vi "Edit WaitMoniter.vi"(8 "error in":errorcluster, 10 "WaitMoniter Input":T2={"Wait Time(S)"=10.0, "Chamber Temp(Deg C)"=10.0, "Chamber Temp Tolerance(%)"=10.0, "RMS Current(A)"=10.0, "RMS Current Tolerance(%)"=10.0, "Temperature Control"=FALSE, "RMS Control"=FALSE, "RMS Current Min(A)"=10.0, "RMS Current Max(A)"=10.0, "Chamber Temp Min(Deg C)"=10.0, "Chamber Temp Max(Deg C)"=10.0, "HVPPS Current Max(A)"=10.0, "HVPPS Control"=FALSE, "HVPPS Current(A)"=10.0} {"HVPPS Current(A)" format="%#_13g"; "HVPPS Current Max(A)" format="%#_13g"; "Chamber Temp Max(Deg C)" format="%#_13g"; "Chamber Temp Min(Deg C)" format="%#_13g"; "RMS Current Max(A)" format="%#_13g"; "RMS Current Min(A)" format="%#_13g"; "RMS Current Tolerance(%)" format="%#_13g"; "RMS Current(A)" format="%#_13g"; "Chamber Temp Tolerance(%)" format="%#_13g"; "Chamber Temp(Deg C)" format="%#_13g"; "Wait Time(S)" format="%#_13g"}, 11 "Sequence Context In":refnum<k7>) -> (0 "error out":errorcluster, 2 "WaitMoniter Output":T2={"Wait Time(S)"=10.0, "Chamber Temp(Deg C)"=10.0, "Chamber Temp Tolerance(%)"=10.0, "RMS Current(A)"=10.0, "RMS Current Tolerance(%)"=10.0, "Temperature Control"=FALSE, "RMS Control"=FALSE, "RMS Current Min(A)"=10.0, "RMS Current Max(A)"=10.0, "Chamber Temp Min(Deg C)"=10.0, "Chamber Temp Max(Deg C)"=10.0, "HVPPS Current Max(A)"=10.0, "HVPPS Control"=FALSE, "HVPPS Current(A)"=10.0} {"HVPPS Current(A)" format="%#_13g"; "HVPPS Current Max(A)" format="%#_13g"; "Chamber Temp Max(Deg C)" format="%#_13g"; "Chamber Temp Min(Deg C)" format="%#_13g"; "RMS Current Max(A)" format="%#_13g"; "RMS Current Min(A)" format="%#_13g"; "RMS Current Tolerance(%)" format="%#_13g"; "RMS Current(A)" format="%#_13g"; "Chamber Temp Tolerance(%)" format="%#_13g"; "Chamber Temp(Deg C)" format="%#_13g"; "Wait Time(S)" format="%#_13g"})   [LabVIEW 2023, in "LTT_TeststandSteptypes.lvlib"]
uses:
  LTT_TeststandSteptypes.lvlib
  Control/Wait Monitor Control.ctl
  Control/Moniter Step Control.ctl
  <vilib>/addons/TestStand/_TSUtility.llb/TestStand - Start Modal Dialog (Sequence Context).vi
  <vilib>/addons/TestStand/_TSUtility.llb/TestStand - End Modal Dialog (Sequence Context).vi
  HardwareAbstractionLayer_LVOOP/Database/Database.lvclass
  HardwareAbstractionLayer_LVOOP/Database/SQL Public VI/Control/DB Options.ctl
  HardwareAbstractionLayer_LVOOP/Power Moniter/Wait Monitor_class/Wait Monitor.lvclass
panel:
  in  "WaitMoniter":T1={"Wait Time(S)"=10.0, "RMS Current Min(A)"=10.0, "Temperature Control"=FALSE, "RMS Control"=FALSE, "RMS Current Max(A)"=10.0, "Chamber Temp Min(Deg C)"=10.0, "Chamber Temp Max(Deg C)"=10.0} {"Chamber Temp Max(Deg C)" format="%#_13g"; "Chamber Temp Min(Deg C)" format="%#_13g"; "RMS Current Max(A)" format="%#_13g"; "RMS Current Min(A)" format="%#_13g"; "Wait Time(S)" format="%#_13g"}
  in  "Close":bool
  in  "OK":bool
  # "WAIT AND MONITOR"
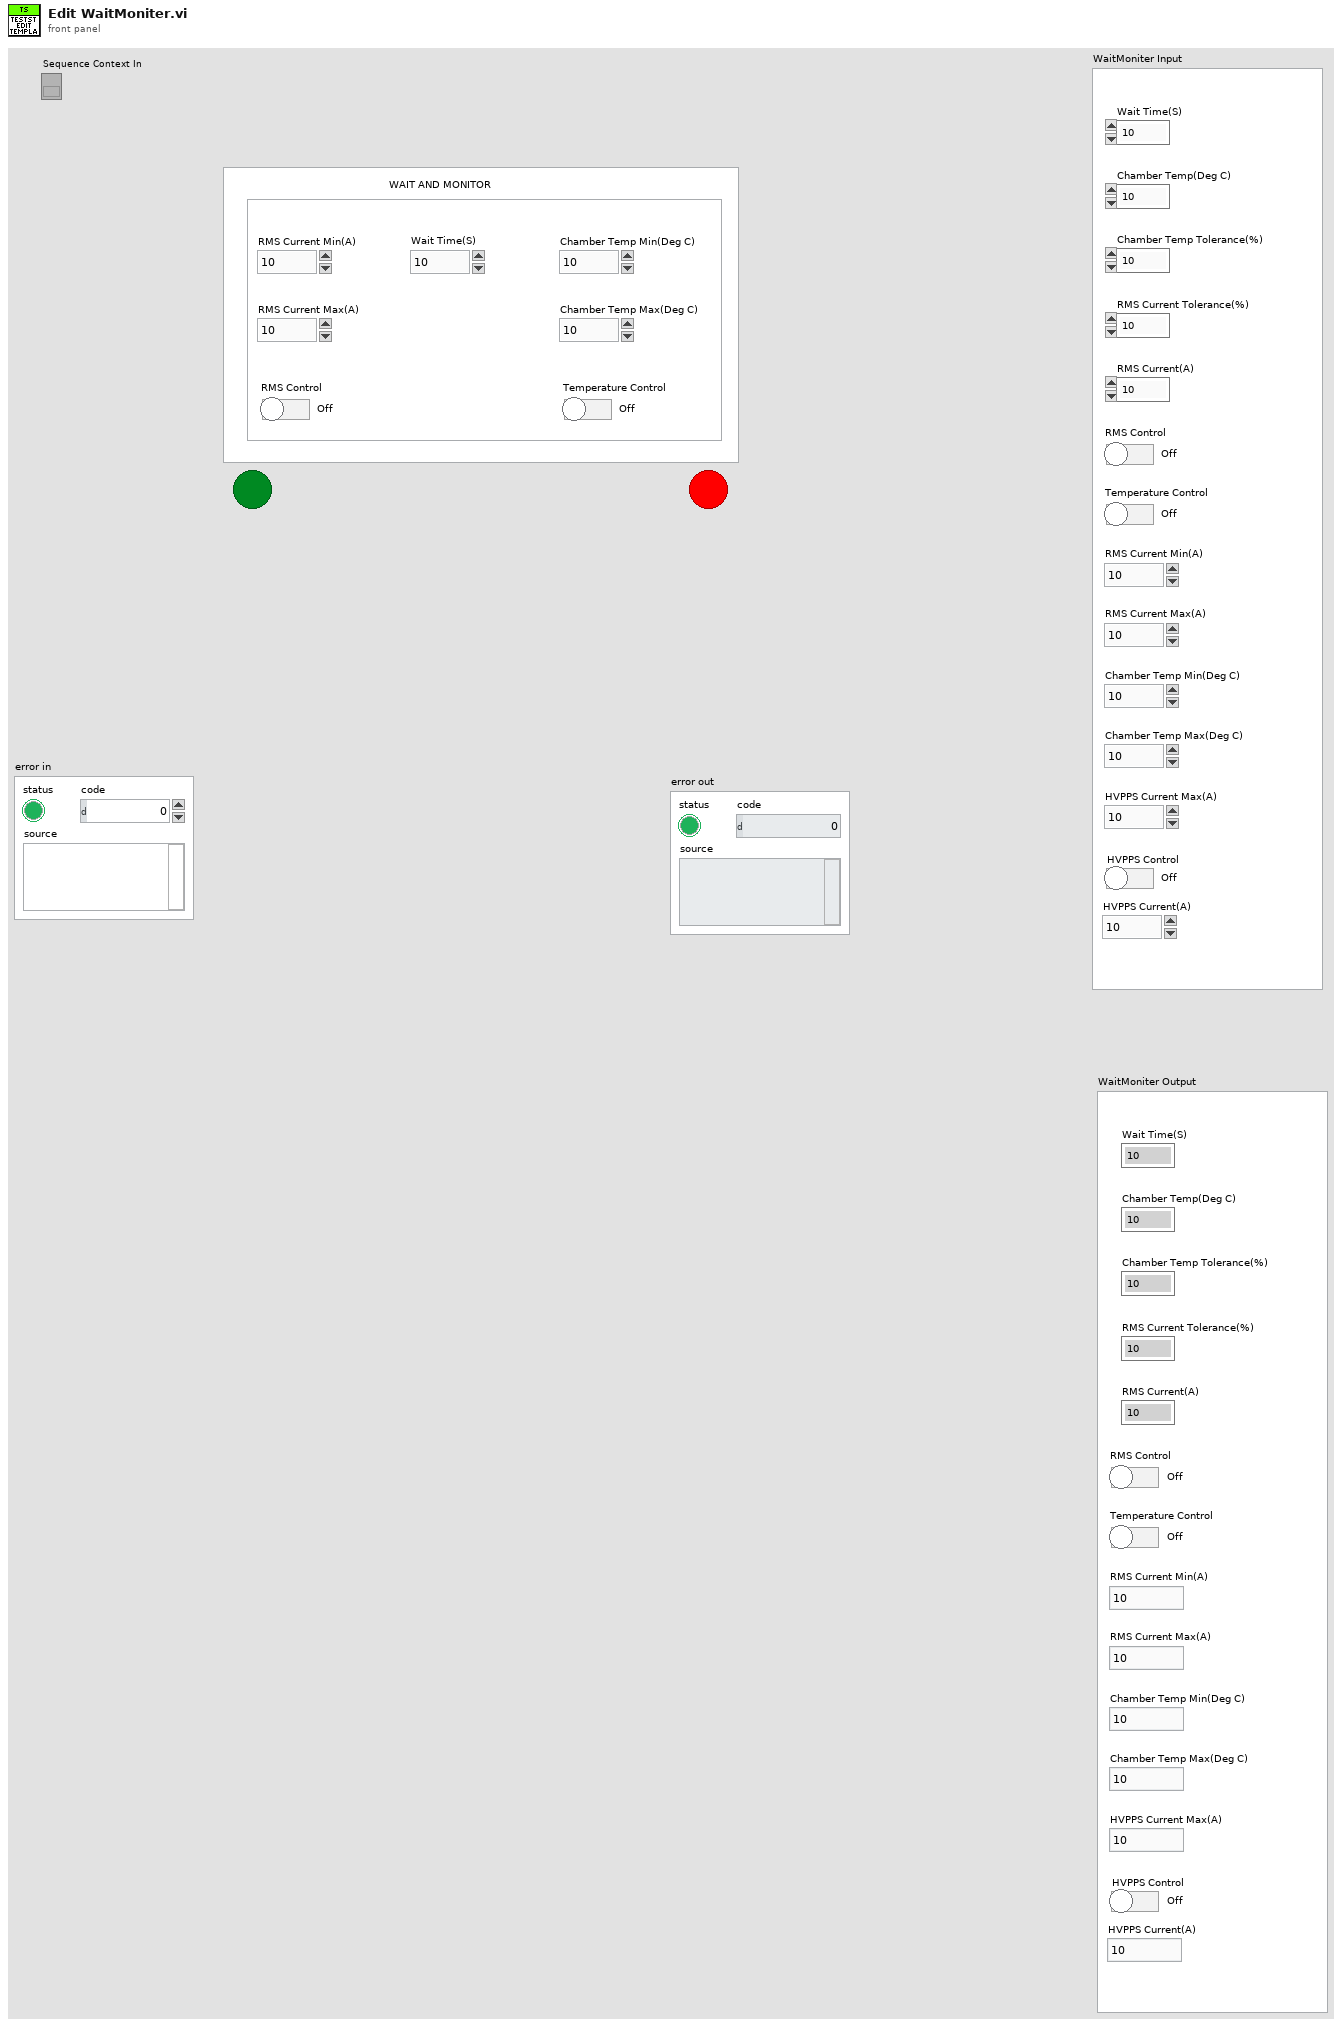
[diagram p1: front panel]
types:
  T1 = typedef "LTT_TeststandSteptypes.lvlib/Wait Monitor Control.ctl" = cluster{"Wait Time(S)":dbl, "RMS Current Min(A)":dbl, "Temperature Control":bool, "RMS Control":bool, "RMS Current Max(A)":dbl, "Chamber Temp Min(Deg C)":dbl, "Chamber Temp Max(Deg C)":dbl}
  T2 = typedef "HardwareAbstractionLayer_LVOOP.lvlib/Wait Monitor.lvclass/Moniter Step Control.ctl" = cluster{"Wait Time(S)":dbl, "Chamber Temp(Deg C)":dbl, "Chamber Temp Tolerance(%)":dbl, "RMS Current(A)":dbl, "RMS Current Tolerance(%)":dbl, "Temperature Control":bool, "RMS Control":bool, "RMS Current Min(A)":dbl, "RMS Current Max(A)":dbl, "Chamber Temp Min(Deg C)":dbl, "Chamber Temp Max(Deg C)":dbl, "HVPPS Current Max(A)":dbl, "HVPPS Control":bool, "HVPPS Current(A)":dbl}
  T3 = typedef "HardwareAbstractionLayer_LVOOP.lvlib/Database.lvclass/DB Options.ctl" = enum16{"Init", "Select Data", "Insert Data", "Update Data", "Delete Data", "Execute Query", "Create Schema", "Create Table", "List Tables", "List Columns", "Close"}
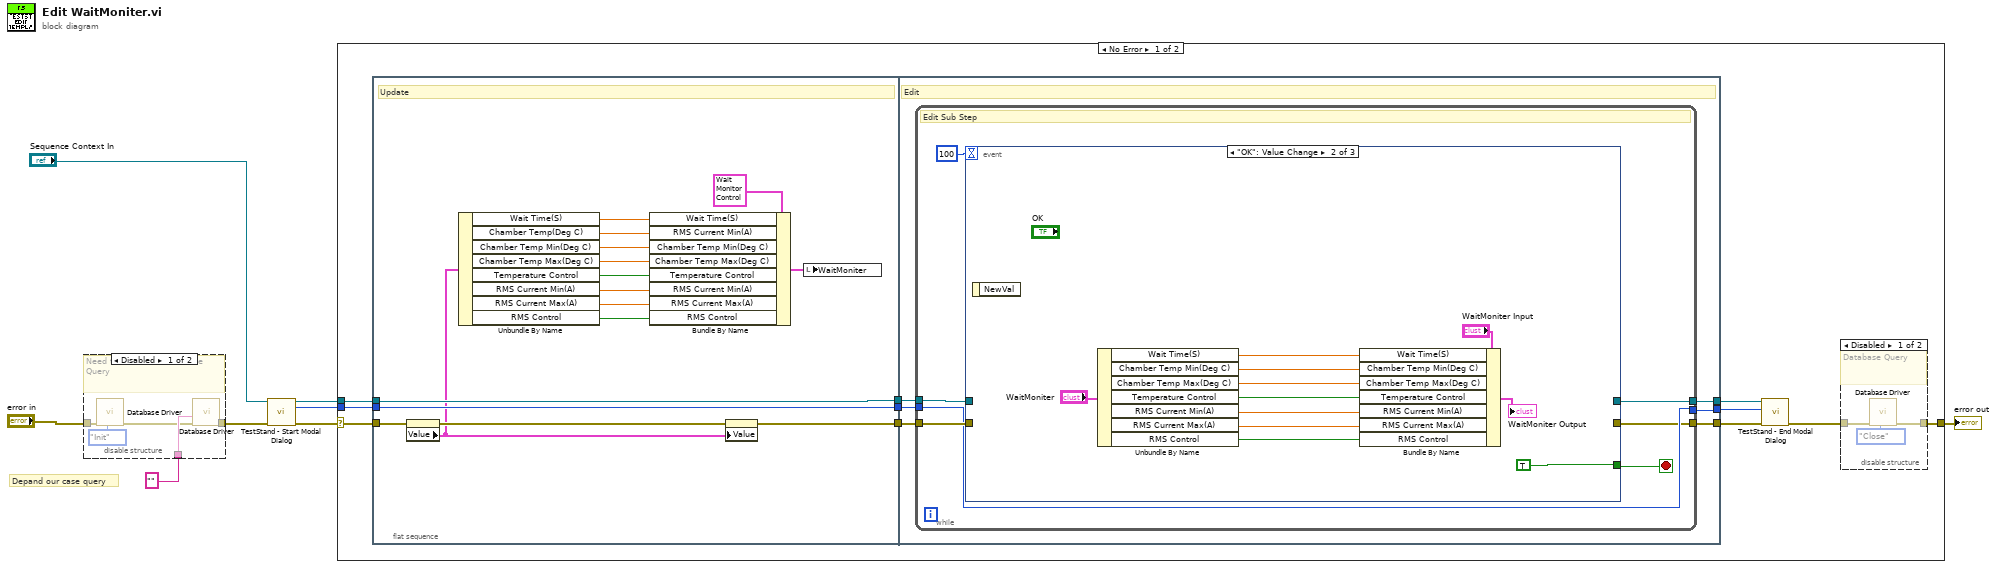
[diagram p0: block diagram]
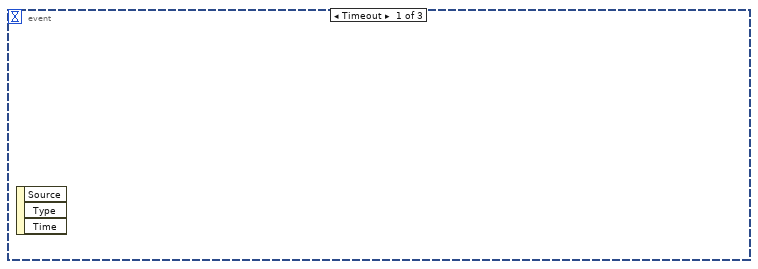
[diagram p3: hidden frame]
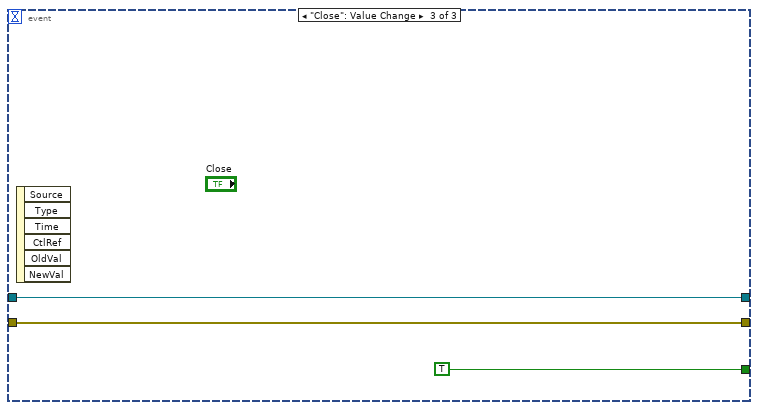
[diagram p4: hidden frame]
diagram:
  # "Depand our case query"
  n1 = disable-structure shown="Disabled" {
    disable-tunnel: "error in" -> [w13 w14]
    disable-tunnel: [w12 w14] -> w4
    disable-tunnel: "" ("SQL query") -> [w11 _]
    frame Disabled {
      # "Need to Enable for Database Query"
      n2 = call "Database Driver.vi"("Options"=DB_Options."Init", "error in"=w13) -> ("error out"=w10:errorcluster)  [unwired: 6 in, 3 out]
      n3 = call "Database Driver.vi"("error in"=w10, "SQL query"=w11) -> ("error out"=w12:errorcluster)  [unwired: 6 in, 3 out]
    }
    frame Enabled {
    }
  }
  n4 = call-poly <vilib>:"TestStand - Start Modal Dialog.vi"("Sequence Context In"="Sequence Context In", "error in (no error)"=w4) -> ("Sequence Context Out"=w6:refnum<k7>, "Modal ID"=w5:i32, "error out"=w7:errorcluster)  [unwired: 9 in, 2 out]
  n5 = case shown="No Error" w7 {
    selector: w7 -> [w22 w72]
    tunnel: w6 -> [w19 _]
    tunnel: w5 -> [w18 _]
    tunnel: [w15 w72] -> w2
    frame No Error {
      n6 = flat-sequence {
        tunnel: w22 -> [w42]
        tunnel: [w40] -> w25
        tunnel: w19 -> [w44]
        tunnel: w18 -> [w43]
        tunnel: [w44] -> w24
        tunnel: [w43] -> w23
        tunnel: w25 -> [w48]
        tunnel: [w46] -> w21
        tunnel: w24 -> [w50]
        tunnel: w23 -> [w49]
        tunnel: [w47] -> w17
        tunnel: [w45] -> w16
        frame #0 {
          # "Update"
          n7 = property on="WaitMoniter Input" class="Clust (strict)"(error in=w42) -> (error out=w41:errorcluster, "Value"=w39:T2)  [unwired: 1 in, 1 out]
          n8 = Unbundle By Name(w39) -> ("Wait Time(S)"=w31:dbl, "Chamber Temp(Deg C)"=w32:dbl, "Chamber Temp Min(Deg C)"=w33:dbl, "Chamber Temp Max(Deg C)"=w34:dbl, "Temperature Control"=w35:bool, "RMS Current Min(A)"=w36:dbl, "RMS Current Max(A)"=w37:dbl, "RMS Control"=w38:bool)
          n9 = Bundle By Name(cluster=T1 {"Wait Time(S)"=10.0, "RMS Current Min(A)"=10.0, "Temperature Control"=FALSE, "RMS Control"=FALSE, "RMS Current Max(A)"=10.0, "Chamber Temp Min(Deg C)"=10.0, "Chamber Temp Max(Deg C)"=10.0} ("WaitMoniter"), "Wait Time(S)"=w31, "RMS Current Min(A)"=w32, "Chamber Temp Min(Deg C)"=w33, "Chamber Temp Max(Deg C)"=w34, "Temperature Control"=w35, "RMS Current Min(A)"=w36, "RMS Current Max(A)"=w37, "RMS Control"=w38) -> (w30:T1)
          n10 = property on="WaitMoniter Output" class="Clust (strict)"(error in=w41, "Value"=w39) -> (error out=w40:errorcluster)  [unwired: 1 in, 1 out]
          n11 = local write "WaitMoniter"(w30) -> ()
        }
        frame #1 {
          # "Edit"
          n12 = while {
            tunnel: w50 -> [w55]
            tunnel: w49 -> [w52]
            tunnel: w48 -> [w53]
            tunnel: [w54] -> w45
            tunnel: [w52] -> w47
            tunnel: [w51] -> w46
            stop <- w56 stop-if-true
            # "Edit Sub Step"
            n13 = event shown="[1] \"OK\": Value Change" {
              selector: _ -> [_ _ _]
              dyn-events: _ -> [_ _ _]
              timeout: 100 -> [_ _ _]
              tunnel: [_ TRUE TRUE] -> w56
              tunnel: [_ _ w70] -> w54
              tunnel: w55 -> [_ _ w70]
              tunnel: w53 -> [_ _ w69]
              tunnel: [_ _ w69] -> w51
              event Timeout {
                n14 = event-data() -> ()  [unwired: 1 in, 3 out]
              }
              event "OK": Value Change {
                n15 = event-data() -> ()  [unwired: 1 in, 1 out]
                n16 = Unbundle By Name("WaitMoniter") -> ("Wait Time(S)"=w64:dbl, "Chamber Temp Min(Deg C)"=w63:dbl, "Chamber Temp Max(Deg C)"=w62:dbl, "Temperature Control"=w61:bool, "RMS Current Min(A)"=w58:dbl, "RMS Current Max(A)"=w59:dbl, "RMS Control"=w60:bool)
                n17 = Bundle By Name(cluster="WaitMoniter Input", "Wait Time(S)"=w64, "Chamber Temp Min(Deg C)"=w63, "Chamber Temp Max(Deg C)"=w62, "Temperature Control"=w61, "RMS Current Min(A)"=w58, "RMS Current Max(A)"=w59, "RMS Control"=w60) -> (→"WaitMoniter Output":T2)
              }
              event "Close": Value Change {
                n18 = event-data() -> ()  [unwired: 1 in, 6 out]
              }
            }
          }
        }
      }
      n19 = call-poly <vilib>:"TestStand - End Modal Dialog.vi"("Sequence Context In"=w16, "Modal ID"=w17, "error in (no error)"=w21) -> ("error out"=w20:errorcluster)  [unwired: 12 in]
      n20 = disable-structure shown="Disabled" {
        disable-tunnel: w20 -> [w28 _]
        disable-tunnel: [w27 _] -> w15
        frame Disabled {
          # "Need to Enable for Database Query"
          n21 = call "Database Driver.vi"("Options"=DB_Options."Close", "error in"=w28) -> ("error out"=w27:errorcluster)  [unwired: 6 in, 3 out]
        }
        frame Enabled {
        }
      }
    }
    frame Error {
    }
  }
  "error out" <- w2
